vi "Property i Event.vi"() -> ()   [LabVIEW 2013]
panel:
  out "Numeric Event":bool
  out "Timeout":bool
  in  "Num (Val+Sig)":dbl
  in  "Numeric":dbl
  in  "Num (Val)":dbl
  in  "stop":bool
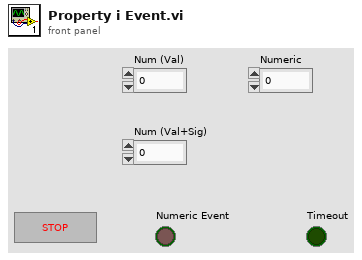
[diagram p1: front panel]
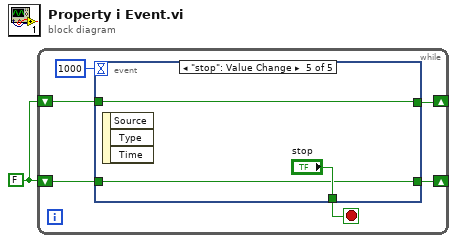
[diagram p0: block diagram]
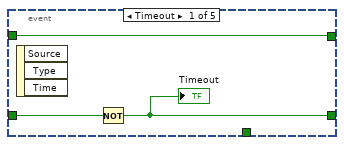
[diagram p2: hidden frame]
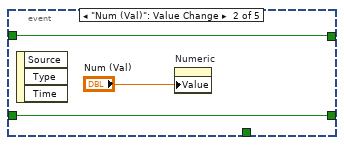
[diagram p3: hidden frame]
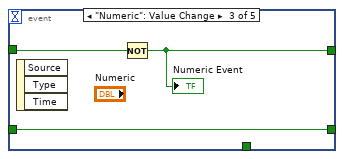
[diagram p4: hidden frame]
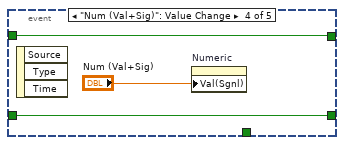
[diagram p5: hidden frame]
diagram:
  w1 = FALSE
  n1 = while {
    shift-right: [w5] -> _
    shift-left: w1 -> [w4]
    shift-right: [w2] -> _
    shift-left: w1 -> [w3]
    stop <- w7 stop-if-true
    n2 = event shown="[4] \"stop\": Value Change" {
      selector: _ -> [_ _ _ _ _]
      dyn-events: _ -> [_ _ _ _ _]
      timeout: 1000 -> [_ _ _ _ _]
      tunnel: [_ _ _ _ "stop"] -> w7
      tunnel: [w9 w13 w16 w19 w21] -> w5
      tunnel: w4 -> [w10 w13 w16 w19 w21]
      tunnel: w3 -> [w8 w11 w15 w18 w20]
      tunnel: [w8 w11 w14 w18 w20] -> w2
      event Timeout {
        n3 = event-data() -> ()  [unwired: 1 in, 3 out]
        n4 = Not(x=w10) -> (.not. x?=w9:bool)
        "Timeout" <- w9
      }
      event "Num (Val)": Value Change {
        n5 = event-data() -> ()  [unwired: 1 in, 3 out]
        n6 = property on="Numeric" class="DigNum (strict)"("Value"="Num (Val)") -> ()  [unwired: 2 in, 2 out]
      }
      event "Numeric": Value Change {
        n7 = event-data() -> ()  [unwired: 1 in, 3 out]
        n8 = Not(x=w15) -> (.not. x?=w14:bool)
        "Numeric Event" <- w14
      }
      event "Num (Val+Sig)": Value Change {
        n9 = event-data() -> ()  [unwired: 1 in, 3 out]
        n10 = property on="Numeric" class="DigNum (strict)"("Val(Sgnl)"="Num (Val+Sig)") -> ()  [unwired: 2 in, 2 out]
      }
      event "stop": Value Change {
        n11 = event-data() -> ()  [unwired: 1 in, 3 out]
      }
    }
  }
